vi "Is Invalid Waveform Element Core.vi"(8 "error in (no error)":errorcluster, 10 "element value (0.0)":dbl format="%.4f", 11 "IVI_Scope in":refnum<class "IVI_Scope.lvclass">) -> (0 "error out":errorcluster, 2 "is invalid":bool, 3 "IVI_Scope out":refnum<class "IVI_Scope.lvclass">)   [LabVIEW 2015, in "IVI_Scope.lvlib" / "IVI_Scope.lvclass"]
doc: "After the read and fetch waveform VIs execute, each element in the waveform array contains either a voltage or a value indicating that the oscilloscope could not sample a voltage. The driver uses an IEEE defined NaN (Not a Number) value to mark as invalid each element in the waveform array for which the oscilloscope could not sample a voltage. This VI determines whether a value you pass from the waveform array is invalid."
uses:
  IVI_Scope.lvclass
  IVI_Scope.lvclass/IVI_Scope.ctl
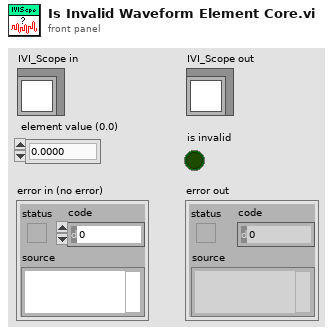
[diagram p1: front panel]
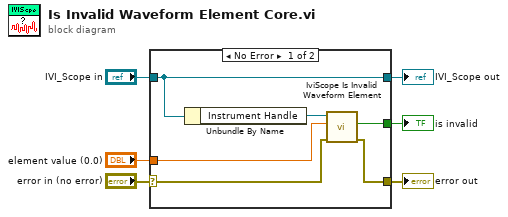
[diagram p0: block diagram]
diagram:
  n1 = case shown="No Error" "error in (no error)" {
    selector: "error in (no error)" -> [w10 w14]
    tunnel: [w9 w14] -> w5
    tunnel: [w12 w13] -> w3
    tunnel: "IVI_Scope in" -> [w12 w13]
    tunnel: "element value (0.0)" -> [w8 _]
    tunnel: [w7 _] -> w1
    frame No Error {
      n2 = Unbundle By Name(w12) -> ("Instrument Handle"=w11:refnum<k15>)
      n3 = call <vilib>:"IviScope Is Invalid Waveform Element.vi"("error in (no error)"=w10, "element value (0.0)"=w8, "instrument handle"=w11) -> ("error out"=w9:errorcluster, "is invalid"=w7:bool)  [unwired: 6 in, 1 out]
    }
    frame Error {
    }
  }
  "error out" <- w5
  "IVI_Scope out" <- w3
  "is invalid" <- w1
